vi "Request State Transition User Event.vi"(8 "error in (no error)":errorcluster, 10 "Message Enqueuer":refnum<class "Message Enqueuer.lvclass">) -> (0 "error out":errorcluster, 1 "State Transition User Event":refnum<user-event>, 2 "Message Enqueuer out":refnum<class "Message Enqueuer.lvclass">)   [LabVIEW 2024, in "State Actor.lvlib" / "State Actor.lvclass"]
uses:
  State Actor.lvclass
  State Actor.lvclass/State Actor.ctl
  State Actor Messages/Get State Transition User Event Msg/Get State Transition User Event Msg.lvclass
  State Transition Event.ctl
  <vilib>/ActorFramework/Message Enqueuer/Message Enqueuer.lvclass
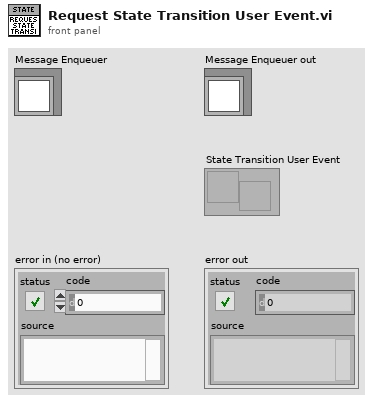
[diagram p1: front panel]
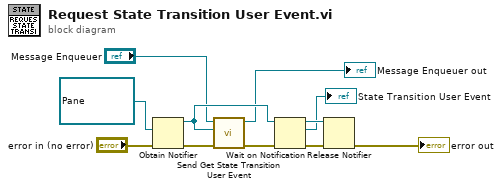
[diagram p0: block diagram]
diagram:
  n1 = Obtain Notifier(notification data type=refnum<user-event> refnum ("State Transition Event"), error in (no error)="error in (no error)") -> (notifier out=w6:refnum<notifier>, error out=w8:errorcluster)  [unwired: 2 in, 1 out]
  n2 = call "Send Get State Transition User Event.vi"("error in (no error)"=w8, "State Transition Event Notifier"=w6, "Message Enqueuer"="Message Enqueuer") -> ("error out"=w11:errorcluster, "Message Enqueuer out"=→"Message Enqueuer out":refnum<class "Message Enqueuer.lvclass">)  [unwired: 7 in]
  n3 = Wait on Notification(notifier=w6, error in (no error)=w11) -> (notifier out=w10:refnum<notifier>, notification=→"State Transition User Event":refnum<user-event>, error out=w9:errorcluster)  [unwired: 2 in, 1 out]
  n4 = Release Notifier(notifier=w10, error in (no error)=w9) -> (error out=→"error out":errorcluster)  [unwired: 1 in, 2 out]
